vi "Text-Replace NaN In Place.vi"(7 "String in":string) -> (8 "String out":string)   [LabVIEW 2020]
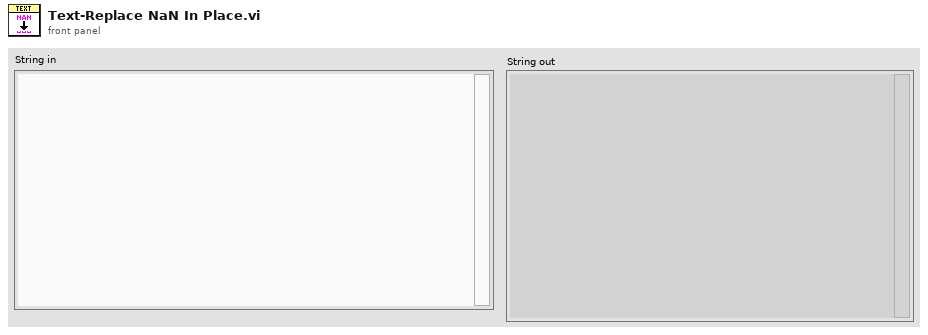
[diagram p1: front panel]
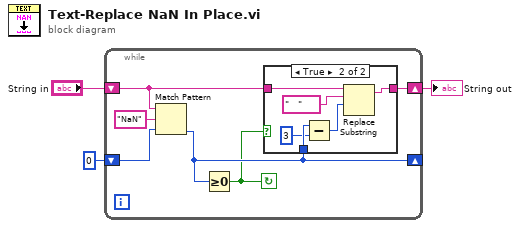
[diagram p0: block diagram]
diagram:
  n1 = while {
    shift-right: [w6] -> w1
    shift-left: "String in" -> [w8]
    shift-right: [w5] -> _
    shift-left: 0 -> [w9]
    stop <- w4 continue-if-true
    n2 = Match Pattern(string=w8, regular expression="NaN", offset (0)=w9) -> (offset past match=w5:i32)  [unwired: 3 out]
    n3 = Greater Or Equal To 0?(x=w5) -> (x >= 0?=w4:bool)
    n4 = case shown="True" w4 {
      tunnel: w8 -> [w10 w16]
      tunnel: [w10 w14] -> w6
      tunnel: w5 -> [_ w13]
      frame False {
      }
      frame True {
        n5 = Subtract(x=w13, y=3) -> (x-y=w11:i32)
        n6 = Replace Substring(3:w11, 4:"   " ("substring (\"\")"), 5:w16) -> (1:w14:string)  [unwired: 1 in, 1 out]
      }
    }
  }
  "String out" <- w1
